vi "Do.vi"(8 "error in (no error)":errorcluster, 9 "Events":refnum<class "Events.lvclass">, 10 "Message Loop Data in":T3, 11 "ISubscribe in":refnum<class "ISubscribe.lvclass">) -> (0 "error out":errorcluster, 1 "Write request":T1, 2 "Message Loop Data out":T3, 3 "ISubscribe out":refnum<class "ISubscribe.lvclass">)   [LabVIEW 2020, in "wamplv.lvlib" / "ISubscribe.lvclass"]
uses:
  ISubscribe.lvclass
  wamplv.lvlib
  WAMP Client/Private/TypeDef/Publish Requests Map.ctl
  WAMP Client/Private/TypeDef/Endpoint Data.ctl
  Call/ICallRequest/ICallRequest.lvclass
  WAMP Client/Private/TypeDef/CALL Request Map.ctl
  WAMP Client/Private/TypeDef/SUBSCRIBE Requests Map.ctl
  WAMP Client/Private/TypeDef/Subscriptions Map.ctl
  WAMP Client/Private/TypeDef/Unsubscribe Requests Map.ctl
  WAMP Client/Private/TypeDef/Unregister requests map.ctl
  WAMP Client/Private/TypeDef/Message Loop Data.ctl
  Events/EventsParent/Events.lvclass
  TypeDefs/Transport type.ctl
  WAMP Client/Private/TypeDef/Write queue item.ctl
  Publish/IPublish/IPublish.lvclass
  Message loop classes/Subscription details/SubscriptionDetailsParent/SubscriptionDetailsParent.lvclass
  Unsubscribe/IUnsubscribe/IUnsubscribe.lvclass
  Register/IRegister/IRegister.lvclass
  Unregister/IUnregister/IUnregister.lvclass
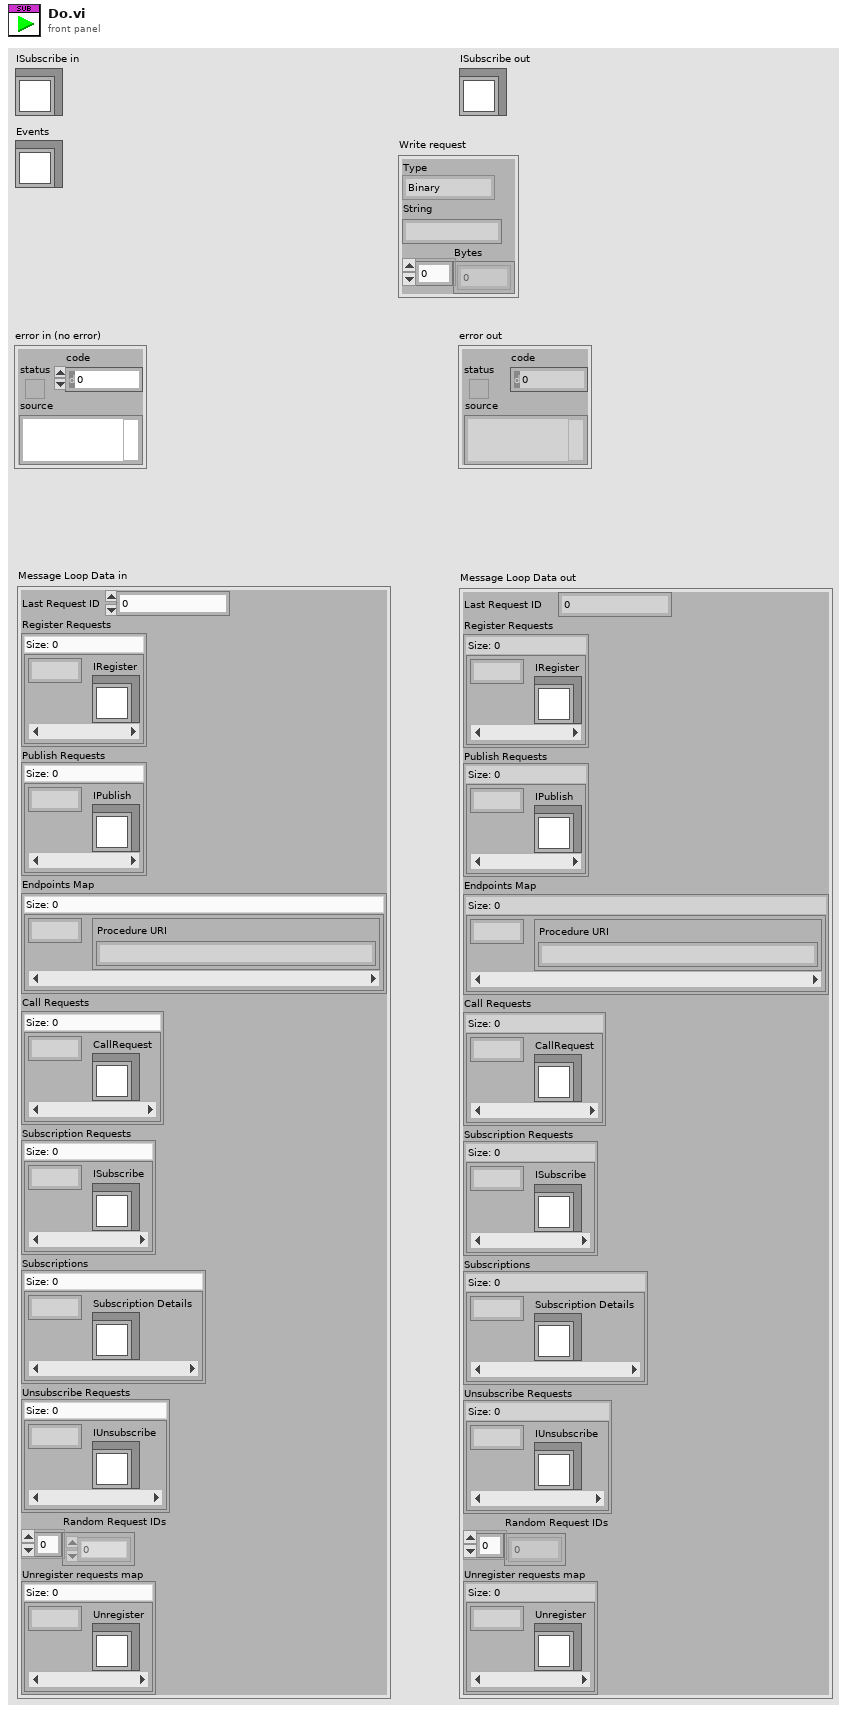
[diagram p1: front panel]
types:
  T1 = typedef "wamplv.lvlib/Write queue item.ctl" = cluster{"Type":T2, "String":string, "Bytes":u8[]}
  T2 = typedef "wamplv.lvlib/Transport type.ctl" = enum16{"Binary", "Text"}
  T3 = typedef "wamplv.lvlib/Message Loop Data.ctl" = cluster{"Last Request ID":u64, "Register Requests":map{u64, refnum<class "IRegister.lvclass">}, "Publish Requests":T4, "Endpoints Map":map{u64, T5}, "Call Requests":T6, "Subscription Requests":T7, "Subscriptions":T8, "Unsubscribe Requests":T9, "Random Request IDs":u64[], "Unregister requests map":T10}
  T4 = typedef "wamplv.lvlib/Publish Requests Map.ctl" = map{u64, refnum<class "IPublish.lvclass">}
  T5 = typedef "wamplv.lvlib/Endpoint Data.ctl" = cluster{"Procedure URI":string}
  T6 = typedef "wamplv.lvlib/CALL Request Map.ctl" = map{u64, refnum<class "ICallRequest.lvclass">}
  T7 = typedef "wamplv.lvlib/SUBSCRIBE Requests Map.ctl" = map{u64, refnum<class "ISubscribe.lvclass">}
  T8 = typedef "wamplv.lvlib/Subscriptions Map.ctl" = map{u64, refnum<class "SubscriptionDetailsParent.lvclass">}
  T9 = typedef "wamplv.lvlib/Unsubscribe Requests Map.ctl" = map{u64, refnum<class "IUnsubscribe.lvclass">}
  T10 = typedef "wamplv.lvlib/Unregister requests map.ctl" = map{u64, refnum<class "IUnregister.lvclass">}
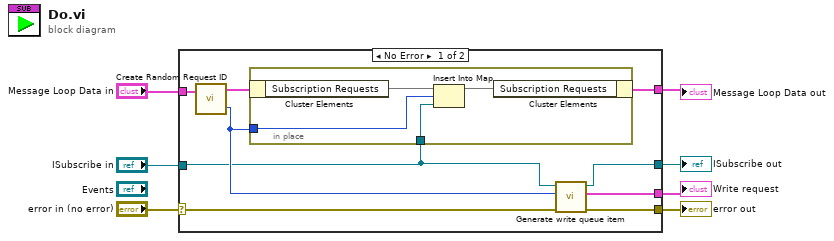
[diagram p0: block diagram]
diagram:
  n1 = case shown="No Error" "error in (no error)" {
    selector: "error in (no error)" -> [w11 w23]
    tunnel: [w10 w23] -> w4
    tunnel: "ISubscribe in" -> [w12 w21]
    tunnel: "Message Loop Data in" -> [w16 w22]
    tunnel: [w14 w22] -> w7
    tunnel: [w9 _] -> w2
    tunnel: [w8 w21] -> w1
    frame No Error {
      n2 = call "Create Random Request ID.vi"("Message Loop Shift Register Data (in)"=w16) -> ("Generated Request ID"=w13:u64, "Message Loop Shift Register Data (out)"=w15:T3)  [unwired: 1 in]
      n3 = in-place "In Place Element Structure" {
        in-place-border: w12 -> [w20]
        in-place-border: w13 -> [w19]
        n4 = in-place-cluster #1(w15) -> ("Subscription Requests"=w18:T7)
        n5 = Insert Into Map(map in=w18, key=w19, value=w20) -> (map out=w17:T7)  [unwired: 2 out]
        n6 = in-place-cluster #1("Subscription Requests"=w17) -> (w14:T3)
      }
      n7 = call-dynamic "Generate write queue item.vi"("error in (no error)"=w11, "Request ID"=w13, "ISubscribe in"=w12) -> ("error out"=w10:errorcluster, "Write queue item"=w9:T1, "ISubscribe out"=w8:refnum<class "ISubscribe.lvclass">)  [unwired: 6 in]
    }
    frame Error {
    }
  }
  "error out" <- w4
  "ISubscribe out" <- w1
  "Message Loop Data out" <- w7
  "Write request" <- w2
